vi "Sample Rate To Ticks.vi"(8 "error in (no error)":errorcluster, 9 "Minimum (S/s)":dbl=1000.0 format="%#_13g", 10 "Maximum (S/s)":dbl=30000.0 format="%#_13g", 11 "Sample Rate (S/s)":dbl) -> (0 "error out":errorcluster, 2 "Actual Sample Rate (S/s)":dbl, 3 "Count (tick/s)":u32)   [LabVIEW 2021]
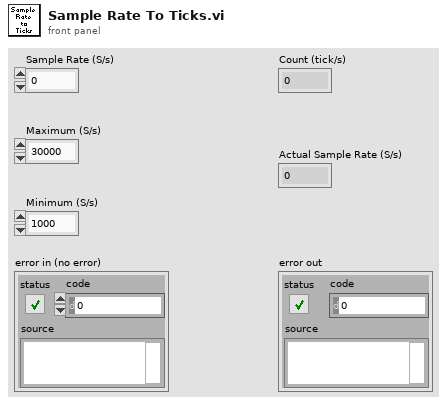
[diagram p1: front panel]
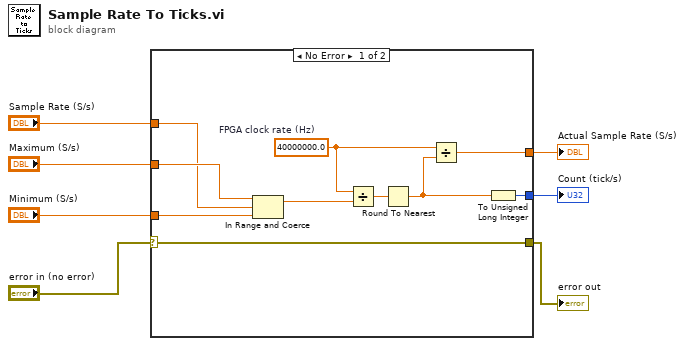
[diagram p0: block diagram]
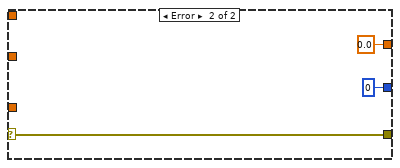
[diagram p2: hidden frame]
diagram:
  n1 = case shown="No Error" "error in (no error)" {
    selector: "error in (no error)" -> [w8 w20]
    tunnel: "Maximum (S/s)" -> [w17 _]
    tunnel: "Minimum (S/s)" -> [w16 _]
    tunnel: "Sample Rate (S/s)" -> [w14 _]
    tunnel: [w13 0.0] -> w4
    tunnel: [w9 u32 0] -> w3
    tunnel: [w8 w20] -> w1
    frame No Error {
      w11 = 40000000.0  # FPGA clock rate (Hz)
      n2 = In Range and Coerce(upper limit=w17, x=w14, lower limit=w16) -> (coerced(x)=w12:dbl)  [unwired: 1 out]
      n3 = Divide(x=w11, y=w12) -> (x/y=w15:dbl)
      n4 = Round To Nearest(number=w15) -> (nearest integer value=w10:dbl)
      n5 = Divide(x=w11, y=w10) -> (x/y=w13:dbl)
      n6 = To Unsigned Long Integer(number=w10) -> (unsigned 32bit integer=w9:u32)
    }
    frame Error {
    }
  }
  "Actual Sample Rate (S/s)" <- w4
  "Count (tick/s)" <- w3
  "error out" <- w1
